vi "POST (Buffer).vi"(6 "timeout":i32=10000, 7 "output file":path, 8 "error in":errorcluster, 9 "buffer":string, 10 "url":string, 11 "http-method in":refnum<class "REST Client.lvclass">) -> (0 "error out":errorcluster, 2 "response":refnum<class "response.lvclass">, 3 "http-method out":refnum<class "REST Client.lvclass">)   [LabVIEW 2020, in "REST Client.lvlib" / "REST Client.lvclass"]
uses:
  REST Client.lvclass
  response/response.lvclass
  http-client/http-client.lvclass
  REST Client.lvclass/REST Client.ctl
  http.lvlib
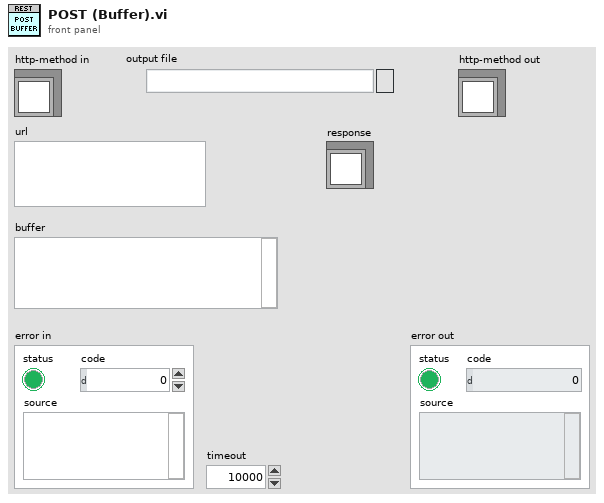
[diagram p1: front panel]
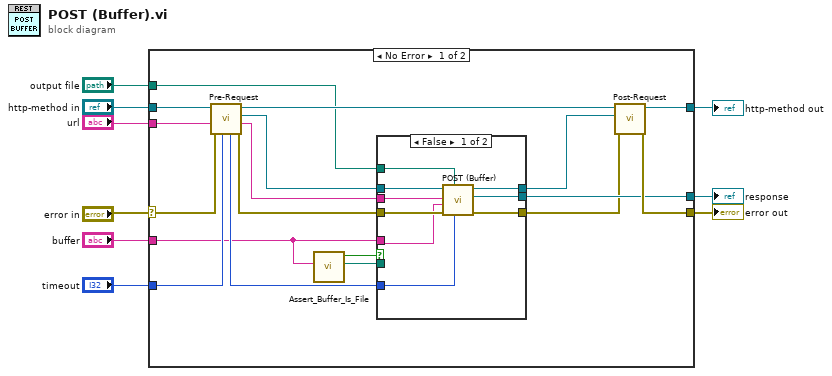
[diagram p0: block diagram]
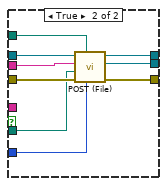
[diagram p2: hidden frame]
diagram:
  n1 = case shown="No Error" "error in" {
    selector: "error in" -> [w26 w47]
    tunnel: [w23 w47] -> w6
    tunnel: [w24 w46] -> w7
    tunnel: "http-method in" -> [w25 w46]
    tunnel: "url" -> [w11 _]
    tunnel: "timeout" -> [w12 _]
    tunnel: "output file" -> [w20 _]
    tunnel: "buffer" -> [w10 _]
    tunnel: [w17 _] -> w1
    frame No Error {
      n2 = call "Pre-Request.vi"("timeout"=w12, "error in (no error)"=w26, "url"=w11, "REST Client in"=w25) -> ("error out"=w14:errorcluster, "Resolved URL"=w15:string, "http-client"=w19:refnum<class "http-client.lvclass">, "REST Client out"=w27:refnum<class "REST Client.lvclass">, "Timeout"=w13:i32)  [unwired: 3 in]
      n3 = call "Assert_Buffer_Is_File.vi"("body"=w10) -> ("File"=w21:path, "is File?"=w22:bool)  [unwired: 9 in]
      n4 = case shown="False" w22 {
        tunnel: w21 -> [_ w37]
        tunnel: w10 -> [w32 _]
        tunnel: w19 -> [w36 w45]
        tunnel: w20 -> [w35 w44]
        tunnel: [w30 w43] -> w18
        tunnel: [w29 w42] -> w17
        tunnel: w13 -> [w28 w41]
        tunnel: w15 -> [w33 w40]
        tunnel: [w31 w39] -> w16
        tunnel: w14 -> [w34 w38]
        frame False {
          n5 = call-dynamic "POST (Buffer).vi"("timeout"=w28, "output file"=w35, "error in"=w34, "buffer"=w32, "url"=w33, "http-method in"=w36) -> ("error out"=w31:errorcluster, "response"=w29:refnum<class "response.lvclass">, "http-method out"=w30:refnum<class "http-client.lvclass">)  [unwired: 3 in]
        }
        frame True {
          n6 = call-dynamic "POST (File).vi"("timeout"=w41, "output file"=w44, "error in"=w38, "file"=w37, "url"=w40, "http-method in"=w45) -> ("error out"=w39:errorcluster, "REST Client.lvlib:response.lvclass"=w42:refnum<class "response.lvclass">, "http-method out"=w43:refnum<class "http-client.lvclass">)  [unwired: 3 in]
        }
      }
      n7 = call "Post-Request.vi"("error in (no error)"=w16, "http-method in"=w18, "REST Client in"=w27) -> ("error out"=w23:errorcluster, "REST Client out"=w24:refnum<class "REST Client.lvclass">)  [unwired: 7 in]
    }
    frame Error {
    }
  }
  "error out" <- w6
  "http-method out" <- w7
  "response" <- w1
